vi "Uart init.vi"(0 "RedPitaya connection in":refnum<k5>, 1 "Baud Rate (9600)":string(combo)="9600", 2 "Bits size (8)":string(combo)="8", 3 "Parity (NONE)":string(combo)="NONE", 4 "Stop bits (1)":string(combo)="1", 5 "error in":errorcluster, 12 "timeout ms (2000)":i32=2000) -> (14 "RedPitaya connection out":refnum<k5>, 19 "error out":errorcluster)   [LabVIEW 2021]
uses:
  Variance measurement/Red_Pitaya/RedPitaya.lvlib
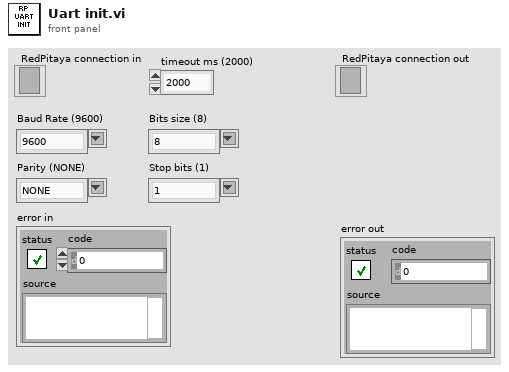
[diagram p1: front panel]
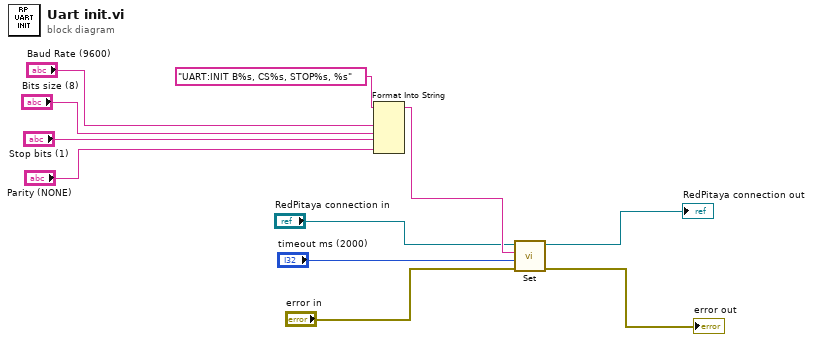
[diagram p0: block diagram]
diagram:
  n1 = Format Into String(format string="UART:INIT B%s, CS%s, STOP%s, %s", "Baud Rate (9600)", "Bits size (8)", "Stop bits (1)", "Parity (NONE)") -> (resulting string=w6:string)  [unwired: 2 in, 1 out]
  n2 = call "Set.vi"("error in"="error in", "timeout ms (2000)"="timeout ms (2000)", "SCPI Message"=w6, "RedPitaya connection in"="RedPitaya connection in") -> ("error out"=→"error out":errorcluster, "RedPitaya connection out"=→"RedPitaya connection out":refnum<k5>)  [unwired: 5 in, 1 out]
